vi "VI Tree.vi"   [LabVIEW 2012, in "Phidget RC Servo.lvlib"]
doc: "${RCServo:VITreeHeader}"
uses:
  <instrlib>/Phidgets/Phidget RC Servo/Phidget RC Servo.lvlib
  <instrlib>/Phidgets/Phidget RC Servo/Public/RCServoStart.vi
  <instrlib>/Phidgets/Phidget RC Servo/Public/RCServoOpen.vi
  <instrlib>/Phidgets/Phidget RC Servo/Public/RCServoClose.vi
panel:
  # "(c) 2015 Phidgets Inc..  ALL RIGHTS RESERVED."
  # "SEE DIAGRAM\nFOR VI TREE."
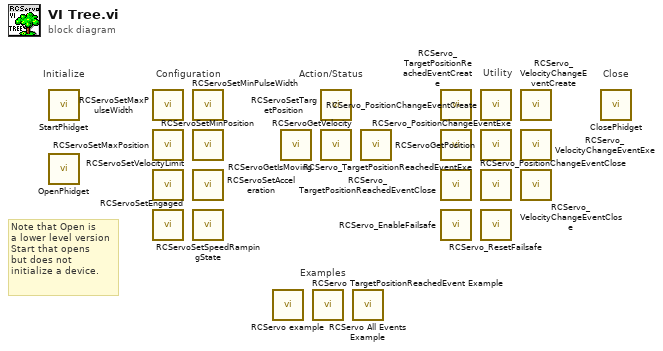
[diagram p0: block diagram]
diagram:
  # "Note that Open is\na lower level version\nStart that opens\nbut does not \ninitialize a device."
  # "Examples"
  # "Configuration"
  # "Utility"
  # "Action/Status"
  # "Close"
  # "Initialize"
  n1 = call-poly <instrlib>:"StartPhidget.vi"() -> ()  [unwired: 12 in, 4 out]
  n2 = call-poly <instrlib>:"OpenPhidget.vi"() -> ()  [unwired: 8 in, 4 out]
  n3 = call <instrlib>:"RCServoSetMaxPulseWidth.vi"() -> ()  [unwired: 9 in, 2 out]
  n4 = call <instrlib>:"RCServoSetMaxPosition.vi"() -> ()  [unwired: 9 in, 2 out]
  n5 = call <instrlib>:"RCServoSetVelocityLimit.vi"() -> ()  [unwired: 9 in, 2 out]
  n6 = call <instrlib>:"RCServoSetEngaged.vi"() -> ()  [unwired: 9 in, 2 out]
  n7 = call <instrlib>:"RCServoSetMinPulseWidth.vi"() -> ()  [unwired: 9 in, 2 out]
  n8 = call <instrlib>:"RCServoSetMinPosition.vi"() -> ()  [unwired: 9 in, 2 out]
  n9 = call <instrlib>:"RCServoSetAcceleration.vi"() -> ()  [unwired: 9 in, 2 out]
  n10 = call <instrlib>:"RCServoSetSpeedRampingState.vi"() -> ()  [unwired: 9 in, 2 out]
  n11 = call <instrlib>:"RCServo example.vi"() -> ()  [unwired: 12 in]
  n12 = call <instrlib>:"RCServoGetIsMoving.vi"() -> ()  [unwired: 8 in, 3 out]
  n13 = call <instrlib>:"RCServo TargetPositionReachedEvent Example.vi"() -> ()  [unwired: 12 in]
  n14 = call <instrlib>:"RCServoSetTargetPosition.vi"() -> ()  [unwired: 9 in, 2 out]
  n15 = call <instrlib>:"RCServoGetVelocity.vi"() -> ()  [unwired: 8 in, 3 out]
  n16 = call <instrlib>:"RCServo All Events Example.vi"() -> ()  [unwired: 12 in]
  n17 = call <instrlib>:"RCServoGetPosition.vi"() -> ()  [unwired: 8 in, 3 out]
  n18 = call <instrlib>:"RCServo_TargetPositionReachedEventCreate.vi"() -> ()  [unwired: 9 in, 3 out]
  n19 = call <instrlib>:"RCServo_TargetPositionReachedEventExe.vi"() -> ()  [unwired: 5 in, 7 out]
  n20 = call <instrlib>:"RCServo_TargetPositionReachedEventClose.vi"() -> ()  [unwired: 10 in, 2 out]
  n21 = call <instrlib>:"RCServo_EnableFailsafe.vi"() -> ()  [unwired: 9 in, 2 out]
  n22 = call <instrlib>:"RCServo_PositionChangeEventCreate.vi"() -> ()  [unwired: 9 in, 3 out]
  n23 = call <instrlib>:"RCServo_PositionChangeEventExe.vi"() -> ()  [unwired: 5 in, 7 out]
  n24 = call <instrlib>:"RCServo_PositionChangeEventClose.vi"() -> ()  [unwired: 10 in, 2 out]
  n25 = call <instrlib>:"RCServo_ResetFailsafe.vi"() -> ()  [unwired: 9 in, 2 out]
  n26 = call <instrlib>:"RCServo_VelocityChangeEventCreate.vi"() -> ()  [unwired: 9 in, 3 out]
  n27 = call <instrlib>:"RCServo_VelocityChangeEventExe.vi"() -> ()  [unwired: 5 in, 7 out]
  n28 = call <instrlib>:"RCServo_VelocityChangeEventClose.vi"() -> ()  [unwired: 10 in, 2 out]
  n29 = call-poly <instrlib>:"ClosePhidget.vi"() -> ()  [unwired: 11 in, 1 out]
